vi "FTW-Endpoint-Multipart-Tell.vi"(0 "FTW Endpoint":refnum<class "FTW-Endpoint-Notifier.lvclass">, 5 "Multipart Message":string[](array[string]), 7 "Timeout":i32 format="%dmsec", 11 "error in":errorcluster) -> (4 "FTW Endpoint out":refnum<class "FTW-Endpoint-Notifier.lvclass">, 6 "Timed out?":bool, 15 "error out":errorcluster)   [LabVIEW 2013, in "FTW-Endpoint-Notifier.lvclass"]
uses:
  FTW-Endpoint-Notifier.lvclass
  FTW-Endpoint-Notifier.lvclass/FTW-Endpoint-Notifier.ctl
panel:
  # "Inputs"
  # "Outputs"
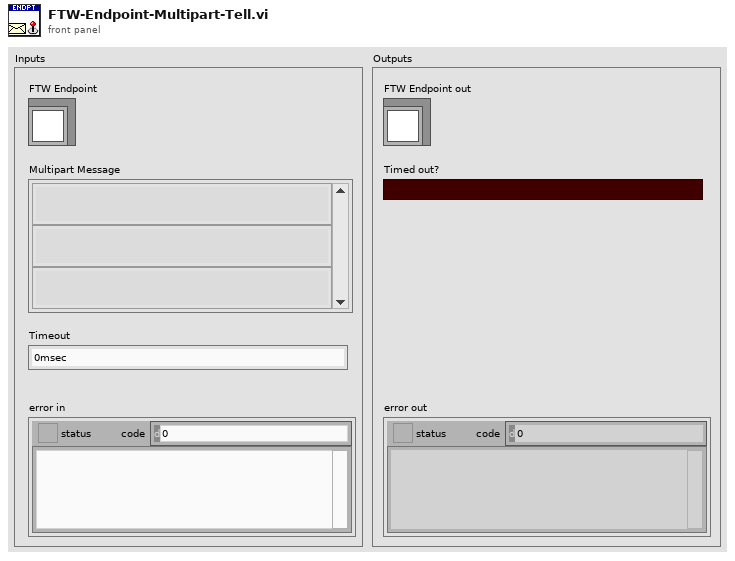
[diagram p1: front panel]
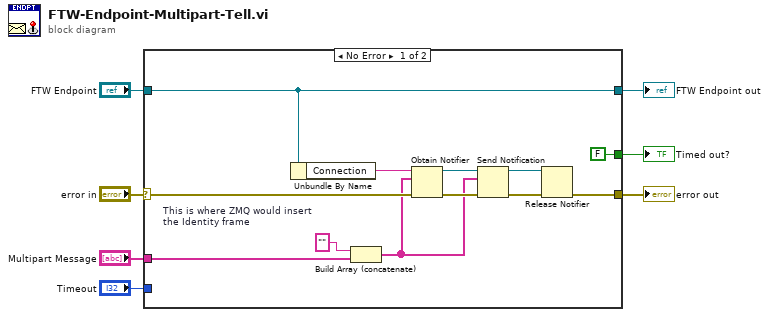
[diagram p0: block diagram]
diagram:
  n1 = case shown="No Error" "error in" {
    selector: "error in" -> [w18 w21]
    tunnel: [w12 w21] -> w7
    tunnel: [w19 w20] -> w5
    tunnel: "FTW Endpoint" -> [w19 w20]
    tunnel: "Multipart Message" -> [w11 _]
    tunnel: [FALSE ("timed out?") _] -> w2
    tunnel: "Timeout" -> [_ _]
    frame No Error {
      w9 = ""  # This is where ZMQ would insert the Identity frame
      n2 = Unbundle By Name(w19) -> ("Connection"=w15:string)
      n3 = Build Array (concatenate)(w9, w11) -> (w10:string[])
      n4 = Obtain Notifier(name (unnamed)=w15, notification data type=w10, error in (no error)=w18) -> (notifier out=w16:refnum<notifier>, error out=w17:errorcluster)  [unwired: 1 in, 1 out]
      n5 = Send Notification(notification=w10, notifier=w16, error in (no error)=w17) -> (notifier out=w14:refnum<notifier>, error out=w13:errorcluster)
      n6 = Release Notifier(notifier=w14, error in (no error)=w13) -> (error out=w12:errorcluster)  [unwired: 1 in, 2 out]
    }
    frame Error {
    }
  }
  "error out" <- w7
  "FTW Endpoint out" <- w5
  "Timed out?" <- w2
